vi "Create Notification Msg.vi"() -> ()   [LabVIEW 2017]
uses:
  <vilib>/Utility/traverseref.llb/TRef TravTarget.ctl
  <vilib>/Utility/traverseref.llb/VI Scripting - Traverse.lvlib
panel:
  out "error out":errorcluster
  in  "Class":path=path "D:/Project/R-Jet/R-Jet/TestVI/Multiple devices Download Tool/Multiple devices Download UI/Multiple devices Download UI/Multiple devices Download UI.lvclass"
  in  "Project":path=path "D:/Project/R-Jet/R-Jet/TestVI/TestVI.lvproj"
  in  "method":path=path "D:/Project/R-Jet/R-Jet/TestVI/Multiple devices Download Tool/Multiple devices Download UI/Multiple devices Download UI/Update Devices List.vi"
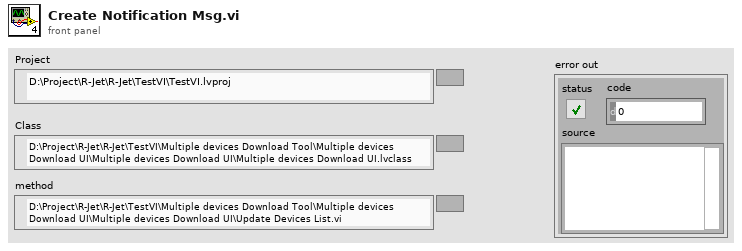
[diagram p1: front panel]
types:
  T1 = typedef "TRef TravTarget.ctl" = enum16{"FP", "BD", "Other"}
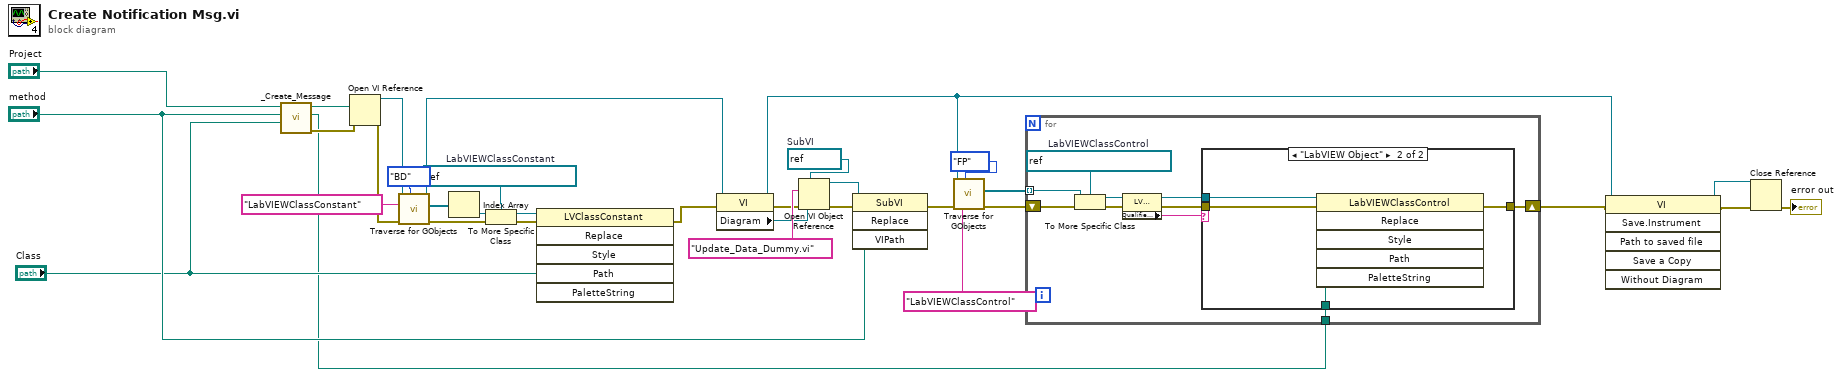
[diagram p0: block diagram]
diagram:
  w15 = refnum<vi> refnum  # SubVI
  w14 = refnum<vi> refnum  # LabVIEWClassConstant
  n1 = call <vilib>:"_Create_Message.vi"("Class"="Class", "Path"="method", "Project Path in"="Project") -> ("error out"=w9:errorcluster, "Msg.lvclass path"=w1:path, "Do path"=w12:path)  [unwired: 6 in]
  n2 = Open VI Reference(vi path=w12, error in (no error)=w9) -> (vi reference=w10:refnum<vi>, error out=w11:errorcluster)  [unwired: 4 in]
  n3 = call <vilib>:"Traverse for GObjects.vi"("Traverse Target"=TRef_TravTarget."BD", "error in (no error)"=w11, "Class Name"="LabVIEWClassConstant", "VI Refnum"=w10) -> ("error out"=w20:errorcluster, "References"=w21:refnum<vi>[], "dup VI Refnum"=w27:refnum<vi>)  [unwired: 4 in, 1 out]
  n4 = Index Array(array=w21) -> (element=w18:refnum<vi>)  [unwired: 1 in]
  n5 = To More Specific Class(target class=w14, reference=w18, error in=w20) -> (specific class reference=w17:refnum<vi>, error out=w19:errorcluster)
  n6 = invoke class="LVClassConstant" method="Replace"(reference=w17, error in=w19, "Path"="Class") -> (error out=w28:errorcluster)  [unwired: 3 in, 5 out]
  n7 = property class="VI"(reference=w27, error in=w28) -> (reference out=w6:refnum<vi>, error out=w22:errorcluster, "Diagram"=w23:refnum<vi>)
  n8 = Open VI Object Reference(7:w15, 8:w22, 10:"Update_Data_Dummy.vi" ("name/order"), 11:w23) -> (0:w25:errorcluster, 3:w24:refnum<vi>)
  n9 = invoke class="SubVI" method="Replace"(reference=w24, error in=w25, "VIPath"="method") -> (error out=w31:errorcluster)  [unwired: 1 in, 3 out]
  n10 = call <vilib>:"Traverse for GObjects.vi"("Traverse Target"=TRef_TravTarget."FP", "error in (no error)"=w31, "Class Name"="LabVIEWClassControl", "VI Refnum"=w6) -> ("error out"=w30:errorcluster, "References"=w29:refnum<vi>[])  [unwired: 4 in, 2 out]
  n11 = for {
    shift-right: [w40] -> w7
    shift-left: w30 -> [w42]
    tunnel: w29 -> [w37] mode=indexing
    tunnel: w1 -> [w35]
    w38 = refnum<vi> refnum  # LabVIEWClassControl
    n12 = To More Specific Class(target class=w38, reference=w37, error in=w42) -> (specific class reference=w43:refnum<vi>, error out=w44:errorcluster)
    n13 = property class="LVClassControl"(reference=w43, error in=w44) -> (reference out=w41:refnum<vi>, error out=w39:errorcluster, "QualifiedName"=w36:string)
    n14 = case shown="\"LabVIEW Object\"" w36 {
      tunnel: w41 -> [_ w49]
      tunnel: [w45 w47] -> w40
      tunnel: w39 -> [w45 w48]
      tunnel: w35 -> [_ w46]
      frame "False", Default {
      }
      frame "LabVIEW Object" {
        n15 = invoke class="LabVIEWClassControl" method="Replace"(reference=w49, error in=w48, "Path"=w46) -> (error out=w47:errorcluster)  [unwired: 3 in, 5 out]
      }
    }
  }
  n16 = invoke class="VI" method="Save.Instrument"(reference=w6, error in=w7) -> (reference out=w5:refnum<vi>, error out=w8:errorcluster)  [unwired: 4 in, 4 out]
  n17 = Close Reference(reference=w5, error in (no error)=w8) -> (error out=→"error out":errorcluster)
